vi "2018新生赛完成版.vi"() -> ()   [LabVIEW 2013]
doc: "本范例根据用户指示，对串口执行读写操作。范例运行时可按下“写入”或“读取”按钮，以及修改“读数”。\n\n设置的串口参数必须匹配连接仪器或设备的参数。本范例中，“读数”参数可指定串口读取的字节数。如端口字节超过指定的字节数，超出部分将不会被读取。如端口字节数少于指定的字节数，将返回超时错误。\n\n本范例可扩展流控制选项以包括XON和XOFF，从而允许用户选择控制字符。同时，用户可启用或禁用中止符。部分设备需要通过终止符确定命令字符串的结束位置。部分设备将发送终止符以说明待读取数据的末端。本范例演示了缓冲区中检测到终止符时，结束“读取”操作或添加终止符至“写入”数据末端的方法。"
uses:
  E:/National Instruments/LabVIEW 2013/examples/Instrument IO/Serial/support/Serial - Settings.ctl
  <vilib>/Instr/_visa.llb/VISA Configure Serial Port (Instr).vi
panel:
  out "L":u8
  out "R":u8
  out "D":u8
  out "R":i16(slide) scale=-255.0..255.0
  out "L":i16(slide) scale=-255.0..255.0
  out "DY":u8
  out "DX":u8
  out "TY":u8
  out "TX":u8
  out "HY":u8
  out "HX":u8
  in  "读取":bool
  out "响应":string
  in  "读数":u32=1000
  in  "VISA资源名称 读取":refnum<visa-resource-name>="COM1"
  in  "串口设置 读取":T1={"波特率"=9600, "数据比特"=8, "奇偶"=enum."None", "停止位"=10, "流控制"=0} {"流控制" items=["无"=0, "XON/XOFF"=1, "RTS/CTS"=2, "DTR/DSR"=4]; "停止位" items=["1.0"=10, "1.5"=15, "2.0"=20]; "数据比特" min=5 max=8 step=1; "波特率" items=["75"=75, "110"=110, "134"=134, "150"=150, "300"=300, "600"=600, "1200"=1200, "1800"=1800, "2400"=2400, "4800"=4800, "7200"=7200, "9600"=9600, "14400"=14400, "19200"=19200, "28800"=28800, "38400"=38400, "56000"=56000, "57600"=57600, "115200"=115200, "128000"=128000, "230400"=230400]}
  in  "终止符时结束读取？":bool=TRUE
  in  "终止符":u8=10 format="%.0x"
  in  "终止符时结束写入？":bool=TRUE
  in  "停止":bool
  out "命令":string="*IDN?"
  in  "写入":bool
  in  "串口设置 写入":T1={"波特率"=9600, "数据比特"=8, "奇偶"=enum."None", "停止位"=10, "流控制"=0} {"流控制" items=["无"=0, "XON/XOFF"=1, "RTS/CTS"=2, "DTR/DSR"=4]; "停止位" items=["1.0"=10, "1.5"=15, "2.0"=20]; "数据比特" min=5 max=8 step=1; "波特率" items=["75"=75, "110"=110, "134"=134, "150"=150, "300"=300, "600"=600, "1200"=1200, "1800"=1800, "2400"=2400, "4800"=4800, "7200"=7200, "9600"=9600, "14400"=14400, "19200"=19200, "28800"=28800, "38400"=38400, "56000"=56000, "57600"=57600, "115200"=115200, "128000"=128000, "230400"=230400]}
  in  "VISA资源名称 写入":refnum<visa-resource-name>="COM1"
  # "概述：演示在循环中使用VISA函数连续写入命令至串口仪器或从串口仪器读取响应。\n要求：NI-VISA驱动程序\n操作步骤：\n1. 运行VI。\n2. 指定命令并单击写入按钮。\n3. 单击读取按钮读取响应。\n4. 单击停止按钮停止VI。"
  # "0xA相当于'\\n'字符，为换行符。"
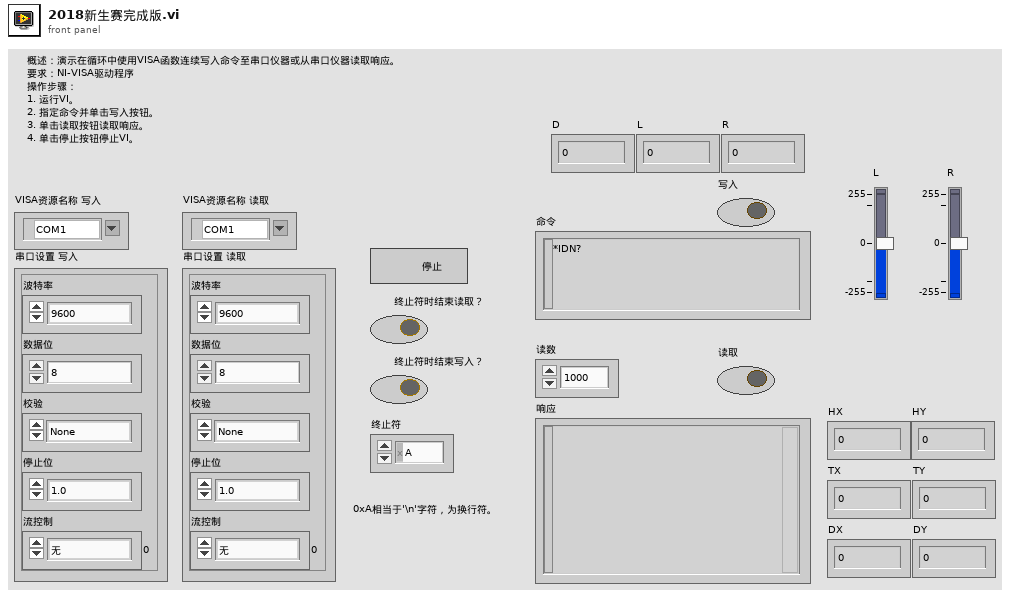
[diagram p1: front panel]
types:
  T1 = typedef "Serial - Settings.ctl" = cluster{"波特率":u32, "数据比特":u16, "奇偶":enum16{"None", "Odd", "Even", "Mark", "Space"}, "停止位":u16, "流控制":u16}
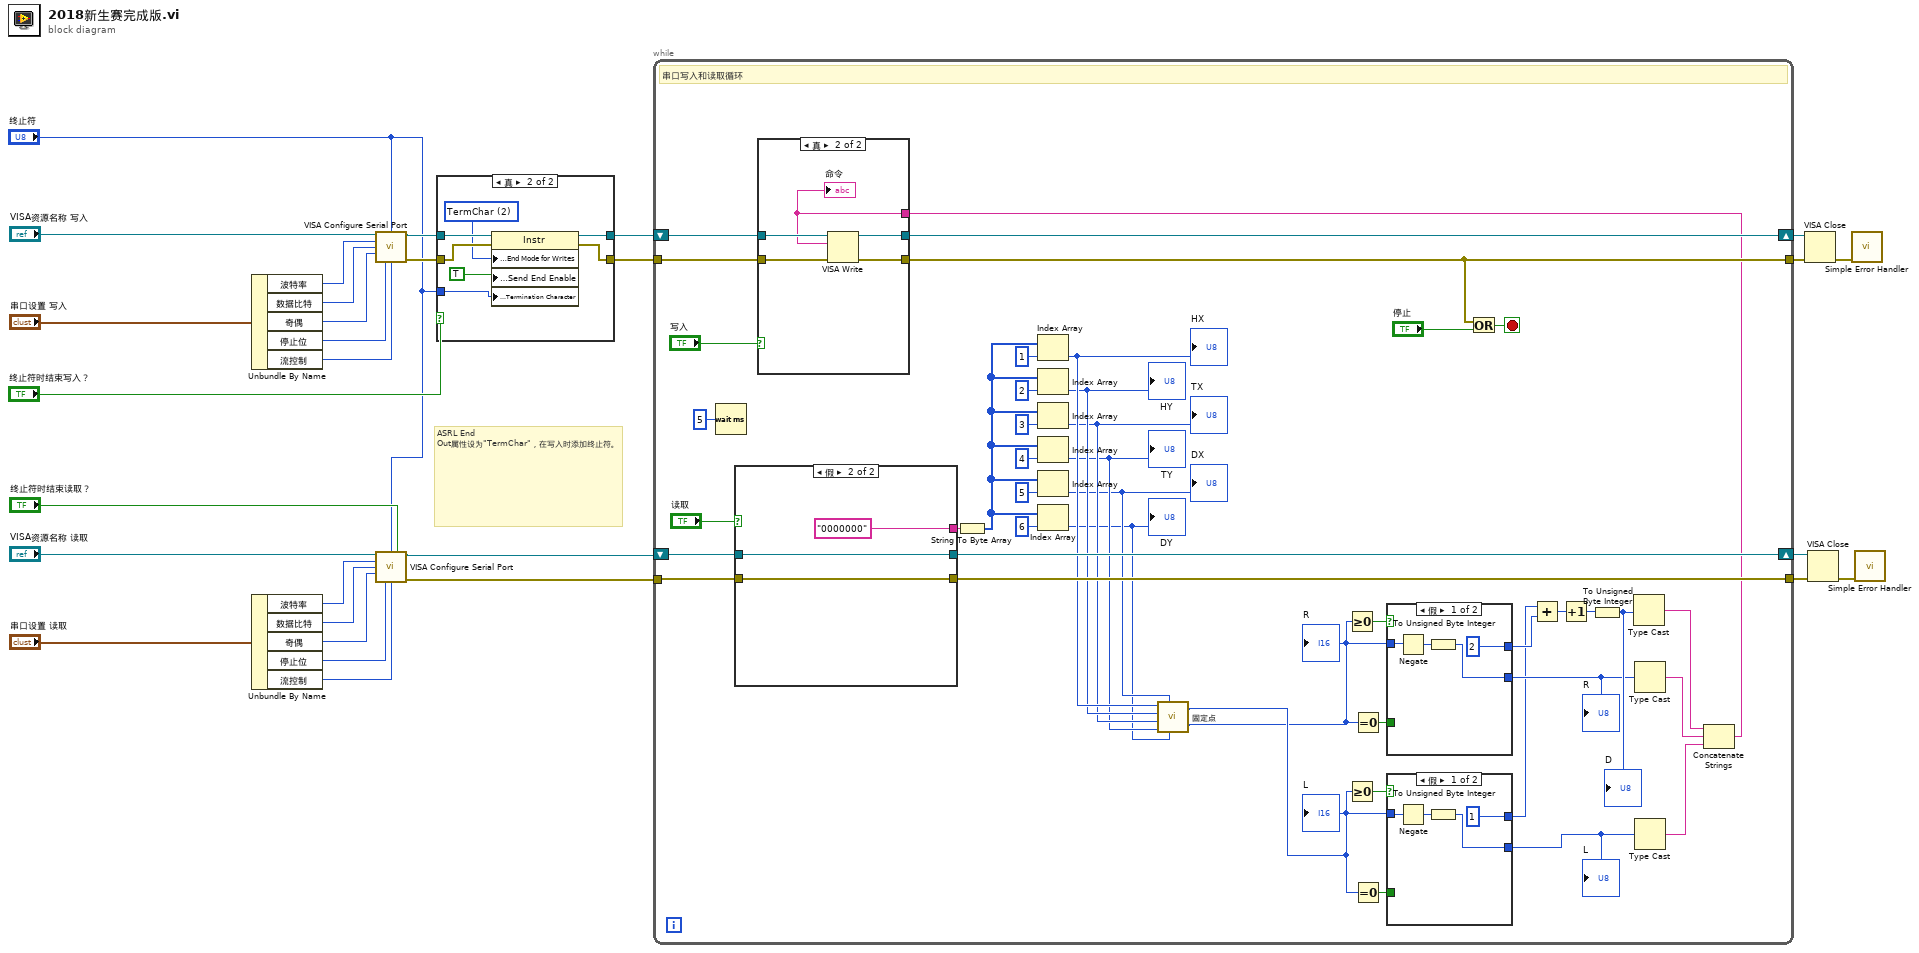
[diagram p0: block diagram]
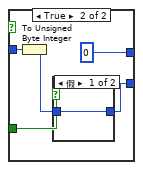
[diagram p3: hidden frame]
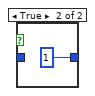
[diagram p4: hidden frame]
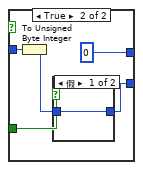
[diagram p5: hidden frame]
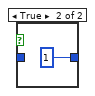
[diagram p6: hidden frame]
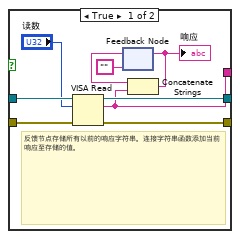
[diagram p7: hidden frame]
diagram:
  # "ASRL End Out属性设为\"TermChar\"，在写入时添加终止符。"
  n1 = Unbundle By Name("串口设置 写入") -> ("波特率"=w25:u32, "数据比特"=w26:u16, "奇偶"=w27:enum16{"None", "Odd", "Even", "Mark", "Space"}, "停止位"=w28:u16, "流控制"=w21:u16)
  n2 = Unbundle By Name("串口设置 读取") -> ("波特率"=w13:u32, "数据比特"=w14:u16, "奇偶"=w15:enum16{"None", "Odd", "Even", "Mark", "Space"}, "停止位"=w16:u16, "流控制"=w9:u16)
  n3 = call-poly "VISA Configure Serial Port"("VISA resource name"="VISA资源名称 写入", "termination char\n(0xA = '\\n' = LF)"="终止符", "baud rate (9600)"=w25, "data bits (8)"=w26, "parity (0:none)"=w27, "stop bits (10: 1 bit)"=w28, "flow control (0:none)"=w21) -> ("VISA resource name out"=w7:refnum<visa-resource-name>, "error out"=w6:errorcluster)  [unwired: 3 in, 4 out]
  n4 = call-poly "VISA Configure Serial Port"("VISA resource name"="VISA资源名称 读取", "termination char\n(0xA = '\\n' = LF)"="终止符", "Enable Termination\nChar (T)"="终止符时结束读取？", "baud rate (9600)"=w13, "data bits (8)"=w14, "parity (0:none)"=w15, "stop bits (10: 1 bit)"=w16, "flow control (0:none)"=w9) -> ("VISA resource name out"=w3:refnum<visa-resource-name>, "error out"=w2:errorcluster)  [unwired: 2 in, 4 out]
  n5 = case shown="真" "终止符时结束写入？" {
    tunnel: w7 -> [w30 w38]
    tunnel: w6 -> [w31 w37]
    tunnel: [w30 w36] -> w19
    tunnel: [w31 w35] -> w20
    tunnel: "终止符" -> [_ w33]
    frame False {
    }
    frame True {
      w34 = u16 2 items=["None", "LastBit", "TermChar", "Break"] ("Serial Settings:Serial End Mode for Writes")
      n6 = property class="Instr"(reference=w38, error in=w37, "Serial Settings:End Mode for Writes"=w34, "Message Based Settings:Send End Enable"=TRUE, "Message Based Settings:Termination Character"=w33) -> (reference out=w36:refnum<visa-resource-name>, error out=w35:errorcluster)
    }
  }
  n7 = while {
    shift-right: [w72] -> w22
    shift-left: w19 -> [w82]
    tunnel: w20 -> [w81]
    tunnel: w2 -> [w73]
    shift-right: [w75] -> w8
    shift-left: w3 -> [w74]
    tunnel: [w71] -> w5
    tunnel: [w70] -> w4
    stop <- w79 stop-if-true
    # "串口写入和读取循环"
    n8 = Wait (ms)(milliseconds to wait=u32 5) -> ()  [unwired: 1 out]
    n9 = case shown="假" "读取" {
      tunnel: [w111 w116] -> w75
      tunnel: w74 -> [w113 w116]
      tunnel: [w109 w115] -> w70
      tunnel: w73 -> [w112 w115]
      tunnel: [w105 "0000000" ("read buffer")] -> w66
      frame True {
        # "反馈节点存储所有以前的响应字符串。连接字符串函数添加当前响应至存储的值。"
        n10 = VISA Read(VISA resource name=w113, byte count="读数", error in (no error)=w112) -> (VISA resource name out=w111:refnum<visa-resource-name>, read buffer=w105:string, error out=w109:errorcluster)  [unwired: 1 out]
        n11 = feedback #1("") -> (w108:string)
        n12 = Concatenate Strings(w108, w105) -> (w106:string)
        "响应" <- w106
        n13 = feedback-in #1(w106) -> ()
      }
      frame False {
      }
    }
    n14 = String To Byte Array(string=w66) -> (unsigned byte array=w65:u8[])
    n15 = Index Array(array=w65, index=1 ("索引")) -> (element=w44:u8)
    "HX" <- w44
    n16 = Index Array(array=w65, index=2 ("索引")) -> (element=w43:u8)
    "HY" <- w43
    n17 = Index Array(array=w65, index=3 ("索引")) -> (element=w42:u8)
    "TX" <- w42
    n18 = Index Array(array=w65, index=4 ("索引")) -> (element=w41:u8)
    "TY" <- w41
    n19 = Index Array(array=w65, index=5 ("索引")) -> (element=w40:u8)
    "DX" <- w40
    n20 = Index Array(array=w65, index=6 ("索引")) -> (element=w39:u8)
    "DY" <- w39
    n21 = call "固定点.vi"("DY"=w39, "DX"=w40, "TY"=w41, "TX"=w42, "HY"=w43, "HX"=w44) -> ("R"=w45:i16, "L"=w46:i16)
    "L" <- w46
    "R" <- w45
    n22 = Greater Or Equal To 0?(x=w45) -> (x >= 0?=w52:bool)
    n23 = Greater Or Equal To 0?(x=w46) -> (x >= 0?=w50:bool)
    n24 = Equal To 0?(x=w45) -> (x = 0?=w51:bool)
    n25 = Equal To 0?(x=w46) -> (x = 0?=w49:bool)
    n26 = case shown="假" w52 {
      tunnel: w45 -> [w97 w101]
      tunnel: [w96 w98] -> w54
      tunnel: [2 0] -> w57
      tunnel: w51 -> [_ w100]
      frame False {
        n27 = Negate(x=w97) -> (-x=w94:i16)
        n28 = To Unsigned Byte Integer(number=w94) -> (unsigned 8bit integer=w96:u8)
      }
      frame True {
        n29 = To Unsigned Byte Integer(number=w101) -> (unsigned 8bit integer=w99:u8)
        n30 = case shown="假" w100 {
          tunnel: w99 -> [w103 _]
          tunnel: [w103 u8 1] -> w98
          frame False {
          }
          frame True {
          }
        }
      }
    }
    "R" <- w54
    n31 = case shown="假" w50 {
      tunnel: [w86 w88] -> w47
      tunnel: [1 0] -> w48
      tunnel: w49 -> [_ w90]
      tunnel: w46 -> [w83 w87]
      frame False {
        n32 = Negate(x=w83) -> (-x=w84:i16)
        n33 = To Unsigned Byte Integer(number=w84) -> (unsigned 8bit integer=w86:u8)
      }
      frame True {
        n34 = To Unsigned Byte Integer(number=w87) -> (unsigned 8bit integer=w89:u8)
        n35 = case shown="假" w90 {
          tunnel: w89 -> [w92 _]
          tunnel: [w92 u8 1] -> w88
          frame False {
          }
          frame True {
          }
        }
      }
    }
    "L" <- w47
    n36 = Add(x=w48, y=w57) -> (x+y=w58:i32)
    n37 = Increment(x=w58) -> (x+1=w56:i32)
    n38 = To Unsigned Byte Integer(number=w56) -> (unsigned 8bit integer=w55:u8)
    "D" <- w55
    n39 = Type Cast(x=w55) -> (*(type *) &x=w69:string)  [unwired: 1 in]
    n40 = Type Cast(x=w54) -> (*(type *) &x=w68:string)  [unwired: 1 in]
    n41 = Type Cast(x=w47) -> (*(type *) &x=w67:string)  [unwired: 1 in]
    n42 = Concatenate Strings(w69, w68, w67) -> (w53:string)
    n43 = case shown="真" "写入" {
      tunnel: w82 -> [w118 w123]
      tunnel: w81 -> [w117 w122]
      tunnel: [w118 w121] -> w72
      tunnel: [w117 w120] -> w71
      tunnel: w53 -> [_ w119]
      frame False {
      }
      frame True {
        n44 = VISA Write(VISA resource name=w123, write buffer=w119, error in (no error)=w122) -> (VISA resource name out=w121:refnum<visa-resource-name>, error out=w120:errorcluster)  [unwired: 1 out]
        "命令" <- w119
      }
    }
    n45 = Or(x=w71, y="停止") -> (x .or. y?=w79:bool)
  }
  n46 = VISA Close(VISA resource name=w22, error in (no error)=w5) -> (error out=w23:errorcluster)
  n47 = VISA Close(VISA resource name=w8, error in (no error)=w4) -> (error out=w10:errorcluster)
  n48 = call <vilib>:"Simple Error Handler.vi"("error in (no error)"=w23) -> ()  [unwired: 1 in, 8 out]
  n49 = call <vilib>:"Simple Error Handler.vi"("error in (no error)"=w10) -> ()  [unwired: 1 in, 8 out]
